vi "Voltech PM1000+ Harmonics Measurement.vi"() -> ()   [LabVIEW 2015]
doc: "The purpose of this vi is to show the basic measurements that PM1000+ can make. The results are returned using the FRD command. This returns the results that are shown on the screen, in the order in which they appear on the screen. As results are selected using comms, the results are added to the bottom of the list, with the exception of harmonics, which always appear at the end of the list."
uses:
  <vilib>/Utility/error.llb/DialogType.ctl
  <instrlib>/Voltech PM1000+/Public/Configure/Configure Measurements (Normal).vi
  <instrlib>/Voltech PM1000+/Voltech PM1000+.lvlib
panel:
  in  "Reset (True)":bool=TRUE
  in  "ID Query (True)":bool=TRUE
  in  "Enable Autozero (True)":bool=TRUE
  in  "Serial Configuration":T1={"Baud Rate"=19200, "Parity"=0, "Data Bits"=8, "Stop Bits"=10, "Flow Control"=2} {"Flow Control" items=["None"=0, "RTS/CTS"=2]; "Stop Bits" items=["1.0"=10]; "Data Bits" items=["8"=8]; "Parity" items=["None"]; "Baud Rate" items=["9600"=9600, "19200"=19200, "38400"=38400]}
  out "Number of Measurements Taken":u32
  in  "Select Mode (Normal)":u16(ring) items=["Normal", "Ballast", "Inrush", "Standby Power", "Integrator"]
  in  "Enable Blanking (True)":bool=TRUE
  in  "Shunt (Internal)":u16(ring) items=["Internal", "External"]
  in  "Freq Source (Voltage)":u16(ring) items=["Voltage", "Current"]
  in  "Measurements":T2={"Voltage Harmonics"={"Range (7)"=7.0, "Sequence (Odd & Even)"=0}, "Current Harmonics"={"Range (7)"=7.0, "Sequence (Odd & Even)"=0}, "Measurements - Normal"=[20, 21]} {"Current Harmonics"."Sequence (Odd & Even)" items=["Odd & Even", "Odd Only"]; "Current Harmonics"."Range (7)" min=1.0 max=50.0 step=1.0; "Voltage Harmonics"."Sequence (Odd & Even)" items=["Odd & Even", "Odd Only"]; "Voltage Harmonics"."Range (7)" min=1.0 max=50.0 step=1.0}
  in  "Fixed/Auto Ranging":T3 {"Volts Ranging (Auto)" items=["Auto", "10Vpk", "46Vpk", "215Vpk", "900Vpk"]; "Amps Ranging (Auto)" items=["Auto", "0.1Apk", "0.4Apk", "1.6Apk", "6.25Apk", "25Apk", "100Apk"]}
  in  "Scaling":T4={"Voltage Sacling (1.0000)"=1.0, "Current Sacling (1.0000)"=1.0} {"Current Sacling (1.0000)" min=1e-06 max=1000000.0 step=1.0 format="%.6f"; "Voltage Sacling (1.0000)" min=1e-06 max=1000000.0 step=1.0 format="%.6f"}
  in  "VISA resource name":refnum<visa-resource-name>
  in  "stop":bool
  out "Parameter":string[](array[string])
  out "Value":dbl[](array[numeric])
  # "(c) 2008-2009 Voltech Instruments.  ALL RIGHTS RESERVED."
  # "Configuration Side"
  # "1. Leave it as default or set up the PM1000+ instruments on the left  \n    \"Configuration Side\".\n2. Press Ctrl+R to run the test.\n3. Press the lower right side \"STOP\" button to stop the test."
  # "1~50"
  # "1~50"
  # "Results Side"
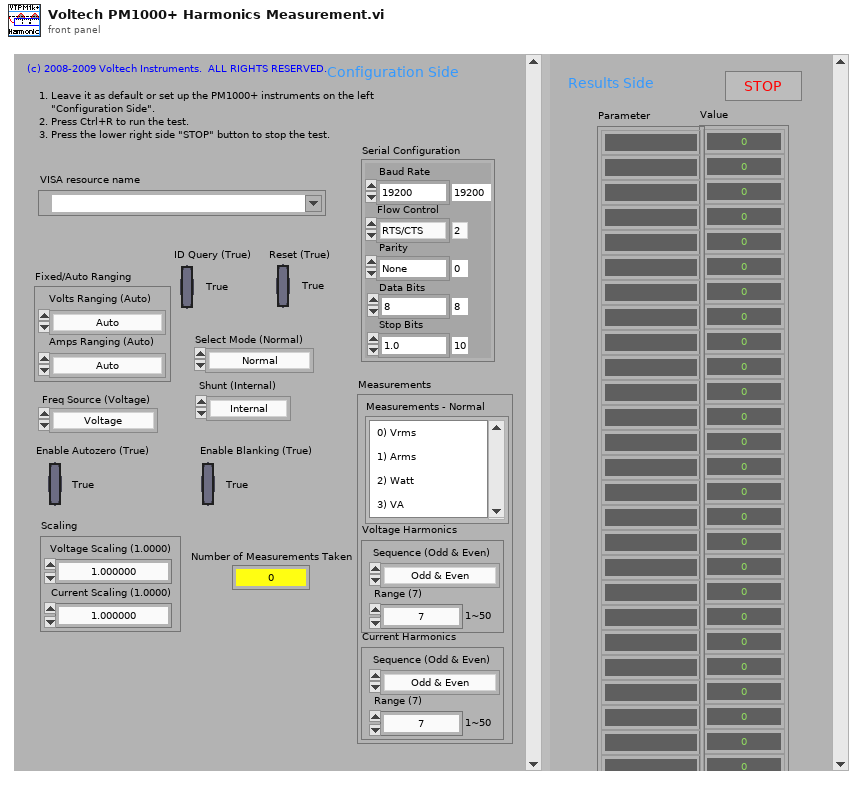
[diagram p1: front panel]
types:
  T1 = cluster{"Baud Rate":u32, "Parity":u16, "Data Bits":u16, "Stop Bits":u16, "Flow Control":u16}
  T2 = cluster{"Voltage Harmonics":cluster{"Range (7)":dbl, "Sequence (Odd & Even)":u16}, "Current Harmonics":cluster{"Range (7)":dbl, "Sequence (Odd & Even)":u16}, "Measurements - Normal":i32[]}
  T3 = cluster{"Amps Ranging (Auto)":u16, "Volts Ranging (Auto)":u16}
  T4 = cluster{"Voltage Sacling (1.0000)":dbl, "Current Sacling (1.0000)":dbl}
  T5 = typedef "DialogType.ctl" = u16
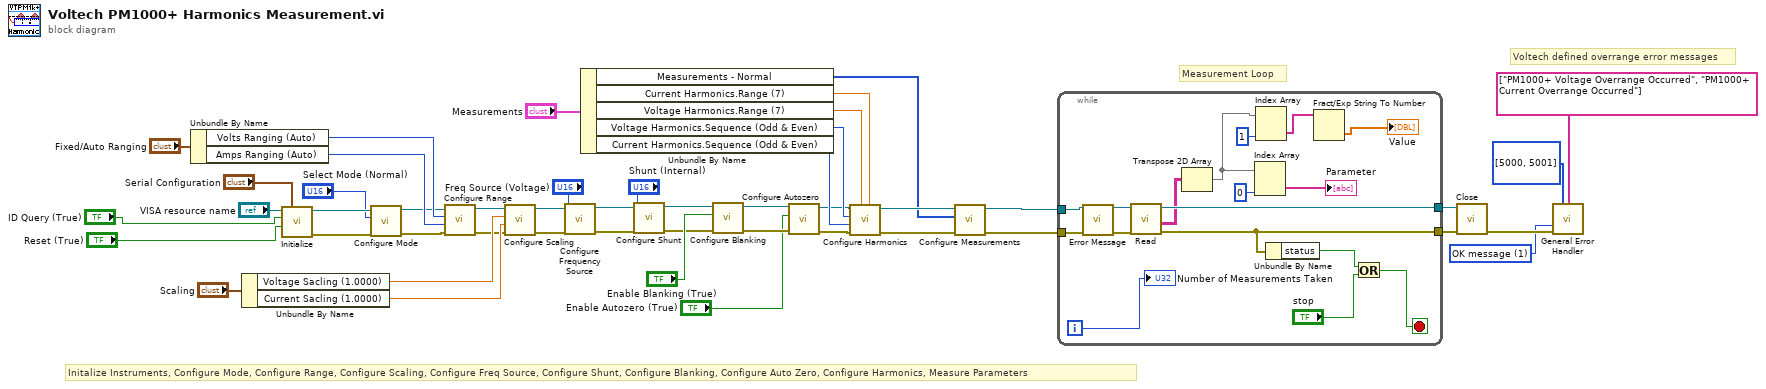
[diagram p0: block diagram]
diagram:
  w15 = T5 1 items=["no dialog", "OK message", "continue or stop message", "OK message + warnings", "continue/stop + warnings"] ("type of dialog (OK msg:1)")
  # "Voltech defined overrange error messages"
  # "Measurement Loop"
  # "Initalize Instruments, Configure Mode, Configure Range, Configure Scaling, Configure Freq Source, Configure Shunt, Configure Blanking, Configure Auto Zero, Configure Harmonics, Measure Parameters"
  n1 = Unbundle By Name("Fixed/Auto Ranging") -> ("Volts Ranging (Auto)"=w38:u16, "Amps Ranging (Auto)"=w37:u16)
  n2 = Unbundle By Name("Scaling") -> ("Voltage Sacling (1.0000)"=w41:dbl, "Current Sacling (1.0000)"=w40:dbl)
  n3 = call <instrlib>:"Initialize.vi"("Serial Configuration"="Serial Configuration", "Reset (True)"="Reset (True)", "ID Query (True)"="ID Query (True)", "VISA resource name"="VISA resource name") -> ("error out"=w7:errorcluster, "VISA resource name out"=w12:refnum<visa-resource-name>)  [unwired: 6 in]
  n4 = call <instrlib>:"Configure Mode.vi"("error in (no error)"=w7, "Select Mode (Normal)"="Select Mode (Normal)", "VISA resource name"=w12) -> ("error out"=w8:errorcluster, "VISA resource name out"=w11:refnum<visa-resource-name>)  [unwired: 7 in]
  n5 = call <instrlib>:"Configure Range.vi"("error in (no error)"=w8, "Current Range (Auto)"=w37, "Voltage Range (Auto)"=w38, "VISA resource name"=w11) -> ("error out"=w9:errorcluster, "VISA resource name out"=w10:refnum<visa-resource-name>)  [unwired: 6 in]
  n6 = call <instrlib>:"Configure Scaling.vi"("error in (no error)"=w9, "Current Sacling (1.0000)"=w40, "Voltage Sacling (1.0000)"=w41, "VISA resource name"=w10) -> ("error out"=w43:errorcluster, "VISA resource name out"=w44:refnum<visa-resource-name>)  [unwired: 6 in]
  n7 = call <instrlib>:"Configure Frequency Source.vi"("error in (no error)"=w43, "Frequency Source (Voltage)"="Freq Source (Voltage)", "VISA resource name"=w44) -> ("error out"=w46:errorcluster, "VISA resource name out"=w45:refnum<visa-resource-name>)  [unwired: 7 in]
  n8 = Unbundle By Name("Measurements") -> ("Measurements - Normal"=w30:i32[], "Current Harmonics.Range (7)"=w34:dbl, "Voltage Harmonics.Range (7)"=w33:dbl, "Voltage Harmonics.Sequence (Odd & Even)"=w29:u16, "Current Harmonics.Sequence (Odd & Even)"=w28:u16)
  n9 = call <instrlib>:"Configure Shunt.vi"("error in (no error)"=w46, "Shunt (Internal)"="Shunt (Internal)", "VISA resource name"=w45) -> ("error out"=w21:errorcluster, "VISA resource name out"=w20:refnum<visa-resource-name>)  [unwired: 7 in]
  n10 = call <instrlib>:"Configure Blanking.vi"("error in (no error)"=w21, "Enable Blanking (True)"="Enable Blanking (True)", "VISA resource name"=w20) -> ("error out"=w18:errorcluster, "VISA resource name out"=w19:refnum<visa-resource-name>)  [unwired: 7 in]
  n11 = call <instrlib>:"Configure Autozero.vi"("error in (no error)"=w18, "Enable Autozero (True)"="Enable Autozero (True)", "VISA resource name"=w19) -> ("error out"=w13:errorcluster, "VISA resource name out"=w14:refnum<visa-resource-name>)  [unwired: 7 in]
  n12 = call <instrlib>:"Configure Harmonics.vi"("Current Harmonic Range (7)"=w34, "Voltage Harmonic Range (7)"=w33, "error in (no error)"=w13, "Current Harmonic Sequence (Odd & Even)"=w28, "Voltage Harmonic Sequence (Odd & Even)"=w29, "VISA resource name"=w14) -> ("error out"=w31:errorcluster, "VISA resource name out"=w32:refnum<visa-resource-name>)  [unwired: 4 in]
  n13 = call-poly <instrlib>:"Configure Measurements.vi"("error in (no error)"=w31, "Normal Measurements"=w30, "VISA resource name"=w32) -> ("error out"=w25:errorcluster, "VISA resource name out"=w26:refnum<visa-resource-name>)  [unwired: 7 in]
  n14 = while {
    tunnel: w26 -> [w53]
    tunnel: w25 -> [w52]
    tunnel: [w64] -> w24
    tunnel: [w51] -> w23
    i -> [w63]
    stop <- w48 stop-if-true
    n15 = call <instrlib>:"Error Message.vi"("VISA resource name"=w53, "error in (no error)"=w52) -> ("VISA resource name out"=w55:refnum<visa-resource-name>, "error out"=w54:errorcluster)  [unwired: 12 in]
    n16 = call <instrlib>:"Read.vi"("error in (no error)"=w54, "VISA resource name"=w55) -> ("error out"=w51:errorcluster, "Measurement Results"=w62:string[][], "VISA resource name out"=w64:refnum<visa-resource-name>)  [unwired: 7 in]
    n17 = Transpose 2D Array(2D array=w62) -> (transposed array=w61:string[][])
    n18 = Index Array(array=w61, index (col)=0) -> (element=→"Parameter":string[])  [unwired: 1 in]
    n19 = Index Array(array=w61, index (col)=1) -> (element=w57:string[])  [unwired: 1 in]
    n20 = Unbundle By Name(w51) -> ("status"=w50:bool)
    n21 = Fract/Exp String To Number(string=w57) -> (number=→"Value":dbl[])  [unwired: 3 in, 1 out]
    n22 = Or(x=w50, y="stop") -> (x .or. y?=w48:bool)
    "Number of Measurements Taken" <- w63
  }
  n23 = call <instrlib>:"Close.vi"("error in (no error)"=w23, "VISA resource name"=w24) -> ("error out"=w16:errorcluster)  [unwired: 9 in]
  n24 = call <vilib>:"General Error Handler.vi"("[user-defined codes]"=i32[] [5000, 5001], "[user-defined descriptions]"=string[] ["PM1000+ Voltage Overrange Occurred", "PM1000+ Current Overrange Occurred"], "type of dialog (OK msg:1)"=w15, "error in (no error)"=w16) -> ()  [unwired: 7 in, 5 out]
